vi "HEWH Solenoid Bank.vi"(0 "VISA session":refnum<visa-resource-name>="MW100", 1 "Valve Bank Setting":T3, 2 "Station ID":T2=enum."A", 5 "Pressurize Tank?":bool, 11 "Error In":errorcluster, 12 "Debug":bool, 13 "Refnum in":T1) -> (4 "dup VISA session":refnum<visa-resource-name>, 15 "Error Out":errorcluster)   [LabVIEW 2016]
uses:
  Type Definitions/HEWH Valve Bank Positions.ctl
  Type Definitions/Station ID Selector.ctl
  Type Definitions/HEWH MW100 Channel Numbers.ctl
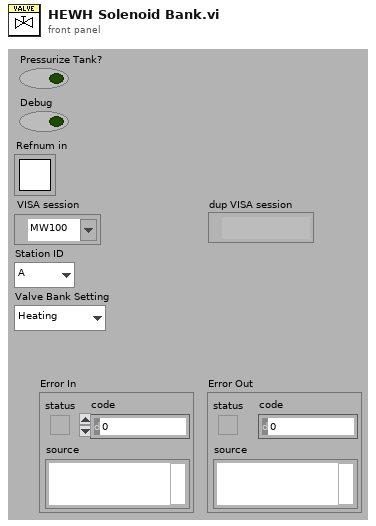
[diagram p1: front panel]
types:
  T1 = typedef "Semaphore RefNum" = refnum<k1>
  T2 = typedef "Station ID Selector.ctl" = enum16{"", "A", "B", "C", "D", "Global"}
  T3 = typedef "HEWH Valve Bank Positions.ctl" = enum16{"Heating", "Purge", "Resting", "Draw"}
  T4 = typedef "HEWH MW100 Channel Numbers.ctl" = string
  T5 = typedef "HEWH Normally Closed Valve Control.ctl" = string
  T6 = typedef "HEWH Normally Open Valve Control.ctl" = string
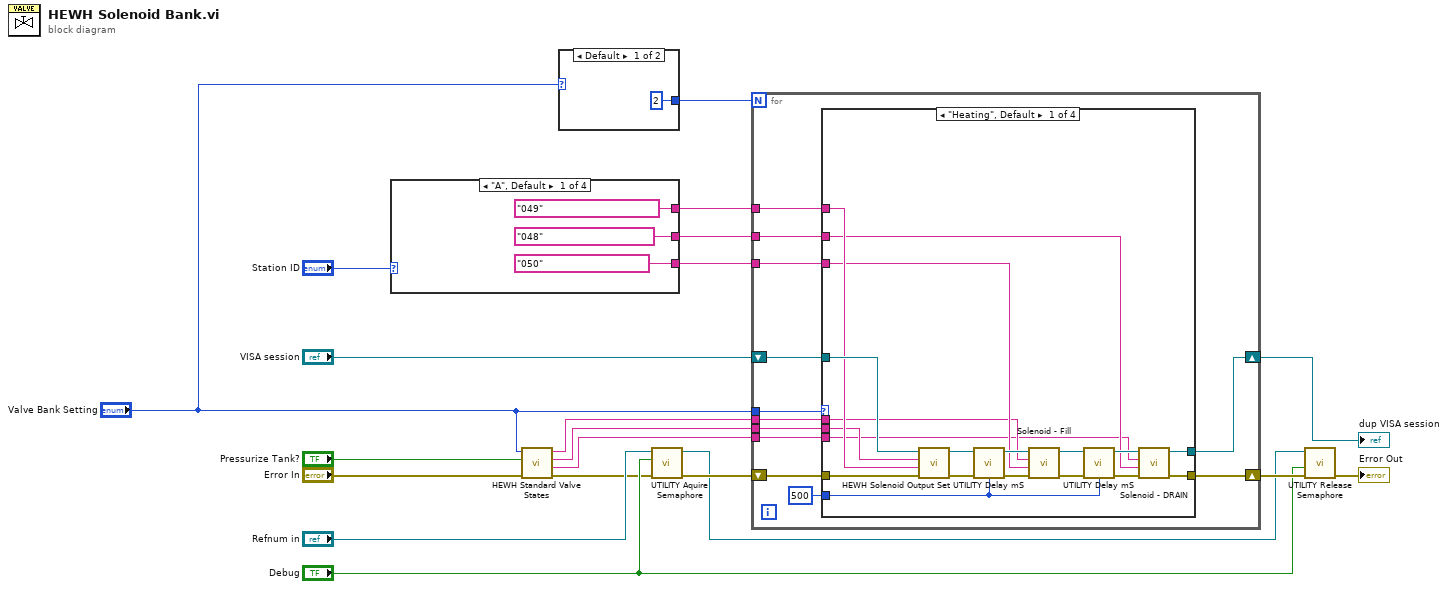
[diagram p0: block diagram]
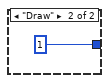
[diagram p2: hidden frame]
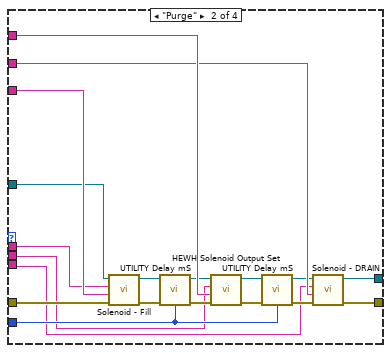
[diagram p3: hidden frame]
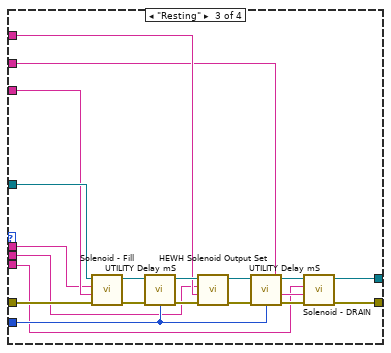
[diagram p4: hidden frame]
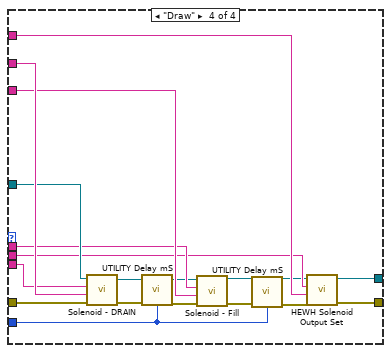
[diagram p5: hidden frame]
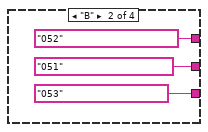
[diagram p6: hidden frame]
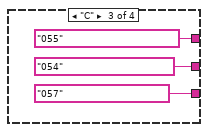
[diagram p7: hidden frame]
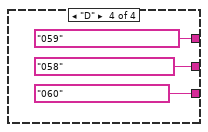
[diagram p8: hidden frame]
diagram:
  n1 = case shown="\"A\", Default" "Station ID" {
    tunnel: [T4 "048" ("HEWH MW100 Channel Numbers") T4 "051" ("HEWH MW100 Channel Numbers") T4 "054" ("HEWH MW100 Channel Numbers") T4 "058" ("HEWH MW100 Channel Numbers")] -> w18
    tunnel: [T4 "049" ("HEWH MW100 Channel Numbers") T4 "052" ("HEWH MW100 Channel Numbers") T4 "055" ("HEWH MW100 Channel Numbers") T4 "059" ("HEWH MW100 Channel Numbers")] -> w20
    tunnel: [T4 "050" ("HEWH MW100 Channel Numbers") T4 "053" ("HEWH MW100 Channel Numbers") T4 "057" ("HEWH MW100 Channel Numbers") T4 "060" ("HEWH MW100 Channel Numbers")] -> w19
    frame "A", Default {
    }
    frame "B" {
    }
    frame "C" {
    }
    frame "D" {
    }
  }
  n2 = call "HEWH Standard Valve States.vi"("Error In"="Error In", "Pressurize Tank?"="Pressurize Tank?", "Valve Bank Setting"="Valve Bank Setting") -> ("Error Out"=w3:errorcluster, "Drain/Purge Valve"=w5:T5, "Outlet Valve"=w6:T6, "Input Valve"=w7:T6)  [unwired: 5 in]
  n3 = case shown="Default" "Valve Bank Setting" {
    tunnel: [2 1] -> w2
    frame Default {
    }
    frame "Draw" {
    }
  }
  n4 = call "UTILITY Aquire Semaphore.vi"("error in (no error)"=w3, "Debug"="Debug", "Refnum in"="Refnum in") -> ("error out"=w12:errorcluster, "Refnum out"=w11:T1)  [unwired: 6 in, 1 out]
  n5 = for {
    N: w2 -> [_]
    tunnel: w20 -> [w46]
    tunnel: w19 -> [w45]
    tunnel: w18 -> [w44]
    tunnel: "Valve Bank Setting" -> [w38]
    tunnel: w7 -> [w37]
    tunnel: w6 -> [w36]
    tunnel: w5 -> [w35]
    shift-right: [w43] -> w17
    shift-left: "VISA session" -> [w42]
    shift-right: [w40] -> w14
    shift-left: w12 -> [w39]
    n6 = case shown="\"Heating\", Default" w38 {
      tunnel: w46 -> [w54 w80 w86 w112]
      tunnel: w45 -> [w53 w79 w87 w111]
      tunnel: w44 -> [w52 w78 w85 w113]
      tunnel: [w50 w71 w89 w101] -> w43
      tunnel: [w62 w70 w88 w103] -> w40
      tunnel: w39 -> [w58 w69 w93 w110]
      tunnel: w42 -> [w57 w68 w92 w109]
      tunnel: w37 -> [w49 w66 w83 w107]
      tunnel: w36 -> [w48 w65 w82 w106]
      tunnel: w35 -> [w47 w64 w81 w108]
      tunnel: u32 500 ("milliseconds to wait") -> [w51 w67 w84 w98]
      frame "Heating", Default {
        n7 = call "HEWH Solenoid Output Set.vi"("Error In"=w58, "HEWH MW100 Channel Numbers"=w54, "Outlet Valve"=w48, "VISA session"=w57) -> ("Error Out"=w61:errorcluster, "dup VISA session"=w56:refnum<visa-resource-name>)  [unwired: 6 in]
        n8 = call "UTILITY Delay mS.vi"("Error In"=w61, "milliseconds to wait"=w51) -> ("Error Out"=w60:errorcluster)  [unwired: 13 in]
        n9 = call "Solenoid - Fill.vi"("Error In"=w60, "HEWH MW100 Channel Numbers"=w53, "Input Valve"=w49, "VISA session"=w56) -> ("Error Out"=w59:errorcluster, "dup VISA session"=w55:refnum<visa-resource-name>)  [unwired: 6 in]
        n10 = call "UTILITY Delay mS.vi"("Error In"=w59, "milliseconds to wait"=w51) -> ("Error Out"=w63:errorcluster)  [unwired: 13 in]
        n11 = call "Solenoid - DRAIN.vi"("Error In"=w63, "HEWH MW100 Channel Numbers"=w52, "Drain/Purge Valve"=w47, "VISA session"=w55) -> ("Error Out"=w62:errorcluster, "dup VISA session"=w50:refnum<visa-resource-name>)  [unwired: 6 in]
      }
      frame "Purge" {
        n12 = call "Solenoid - Fill.vi"("Error In"=w69, "HEWH MW100 Channel Numbers"=w79, "Input Valve"=w66, "VISA session"=w68) -> ("Error Out"=w75:errorcluster, "dup VISA session"=w76:refnum<visa-resource-name>)  [unwired: 6 in]
        n13 = call "UTILITY Delay mS.vi"("Error In"=w75, "milliseconds to wait"=w67) -> ("Error Out"=w74:errorcluster)  [unwired: 13 in]
        n14 = call "HEWH Solenoid Output Set.vi"("Error In"=w74, "HEWH MW100 Channel Numbers"=w80, "Outlet Valve"=w65, "VISA session"=w76) -> ("Error Out"=w73:errorcluster, "dup VISA session"=w77:refnum<visa-resource-name>)  [unwired: 6 in]
        n15 = call "UTILITY Delay mS.vi"("Error In"=w73, "milliseconds to wait"=w67) -> ("Error Out"=w72:errorcluster)  [unwired: 13 in]
        n16 = call "Solenoid - DRAIN.vi"("Error In"=w72, "HEWH MW100 Channel Numbers"=w78, "Drain/Purge Valve"=w64, "VISA session"=w77) -> ("Error Out"=w70:errorcluster, "dup VISA session"=w71:refnum<visa-resource-name>)  [unwired: 6 in]
      }
      frame "Resting" {
        n17 = call "Solenoid - Fill.vi"("Error In"=w93, "HEWH MW100 Channel Numbers"=w87, "Input Valve"=w83, "VISA session"=w92) -> ("Error Out"=w97:errorcluster, "dup VISA session"=w91:refnum<visa-resource-name>)  [unwired: 6 in]
        n18 = call "UTILITY Delay mS.vi"("Error In"=w97, "milliseconds to wait"=w84) -> ("Error Out"=w96:errorcluster)  [unwired: 13 in]
        n19 = call "HEWH Solenoid Output Set.vi"("Error In"=w96, "HEWH MW100 Channel Numbers"=w86, "Outlet Valve"=w82, "VISA session"=w91) -> ("Error Out"=w95:errorcluster, "dup VISA session"=w90:refnum<visa-resource-name>)  [unwired: 6 in]
        n20 = call "UTILITY Delay mS.vi"("Error In"=w95, "milliseconds to wait"=w84) -> ("Error Out"=w94:errorcluster)  [unwired: 13 in]
        n21 = call "Solenoid - DRAIN.vi"("Error In"=w94, "HEWH MW100 Channel Numbers"=w85, "Drain/Purge Valve"=w81, "VISA session"=w90) -> ("Error Out"=w88:errorcluster, "dup VISA session"=w89:refnum<visa-resource-name>)  [unwired: 6 in]
      }
      frame "Draw" {
        n22 = call "Solenoid - DRAIN.vi"("Error In"=w110, "HEWH MW100 Channel Numbers"=w113, "Drain/Purge Valve"=w108, "VISA session"=w109) -> ("Error Out"=w114:errorcluster, "dup VISA session"=w99:refnum<visa-resource-name>)  [unwired: 6 in]
        n23 = call "UTILITY Delay mS.vi"("Error In"=w114, "milliseconds to wait"=w98) -> ("Error Out"=w105:errorcluster)  [unwired: 13 in]
        n24 = call "Solenoid - Fill.vi"("Error In"=w105, "HEWH MW100 Channel Numbers"=w111, "Input Valve"=w107, "VISA session"=w99) -> ("Error Out"=w104:errorcluster, "dup VISA session"=w100:refnum<visa-resource-name>)  [unwired: 6 in]
        n25 = call "UTILITY Delay mS.vi"("Error In"=w104, "milliseconds to wait"=w98) -> ("Error Out"=w102:errorcluster)  [unwired: 13 in]
        n26 = call "HEWH Solenoid Output Set.vi"("Error In"=w102, "HEWH MW100 Channel Numbers"=w112, "Outlet Valve"=w106, "VISA session"=w100) -> ("Error Out"=w103:errorcluster, "dup VISA session"=w101:refnum<visa-resource-name>)  [unwired: 6 in]
      }
    }
  }
  "dup VISA session" <- w17
  n27 = call "UTILITY Release Semaphore.vi"("error in (no error)"=w14, "Debug"="Debug", "Refnum in"=w11) -> ("error out"=→"Error Out":errorcluster)  [unwired: 8 in]
